vi "zapis.vi"() -> ()   [LabVIEW 2020]
panel:
  out "Numeric 2":dbl
  out "Numeric":dbl
  in  "Stop Button":bool
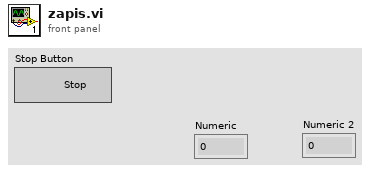
[diagram p1: front panel]
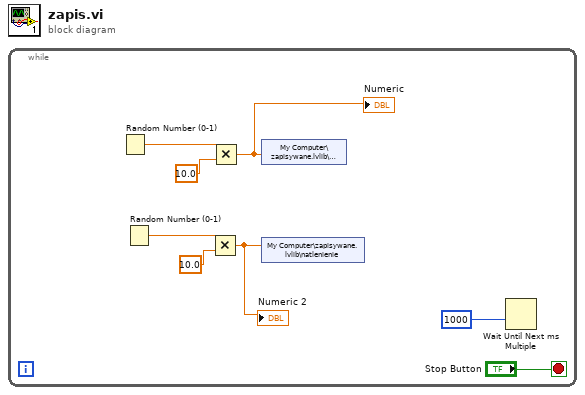
[diagram p0: block diagram]
diagram:
  n1 = while {
    stop <- "Stop Button" stop-if-true
    n2 = Random Number (0-1)() -> (number: 0 to 1=w6:dbl)
    n3 = Random Number (0-1)() -> (number: 0 to 1=w4:dbl)
    n4 = Multiply(x=w4, y=10.0) -> (x*y=w1:dbl)
    "Numeric 2" <- w1
    n5 = Multiply(x=w6, y=10.0) -> (x*y=w2:dbl)
    "Numeric" <- w2
    n6 = shared-variable "My Computer\\zapisywane.lvlib\\poziom"(w2) -> ()  [unwired: 1 in, 1 out]
    n7 = shared-variable "My Computer\\zapisywane.lvlib\\natlenienie"(w1) -> ()  [unwired: 1 in, 1 out]
    n8 = Wait Until Next ms Multiple(millisecond multiple=u32 1000) -> ()  [unwired: 1 out]
  }
